vi "CSConnect.UpdateAllVoltages.vi"(0 "i ref in":refnum<vi>, 2 "In-channel number":i32, 3 "In-Voltage":dbl, 5 "error in (no error)":errorcluster) -> (14 "i ref out":refnum<vi>, 19 "error out":errorcluster)   [LabVIEW 2014, in "CSConnect.lvlib"]
doc: "Updates all voltages. This VI should be executed in ProcCases by the User. The idea is to only the \"Out\"-Voltages that need to be updated.\n\nLicense Agreement for this software:\n\nCopyright (C)\nGesellschaft für Schwerionenforschung, GSI\nPlanckstr. 1\n64291 Darmstadt\nGermany\n\nContact: D.Beck@gsi.de \n\nThis program is free software; you can redistribute it and/or modify it under the terms of the \nGNU General Public License as published by the Free Software Foundation; either version 2 of \nthe license, or (at your option) any later version.\n\nThis program is distributed in the hope that it will be useful, but WITHOUT ANY WARRANTY; \nwithout even the implied warranty of MERCHANTABILITY or FITNESS FOR A PARTICULAR PURPOSE. See the GNU General License for more details (http://www.gnu.org).\n\nGesellschaft für Schwerionenforschung, GSI\nPlanckstr. 1, 64291 Darmstadt, Germany\nFor all questions and ideas contact: M.Richter@gsi.de, H.Brand@gsi.de or D.Beck@gsi.de.\nLast update: 16-JUN-2004"
uses:
  CSConnect.lvlib
  CSCore/CSSystem/CoreLib/CoreLib.int 2 byte array.vi
  CSCore/CSSystem/CoreLib/CoreLib.double 2 byte array.vi
  CSCore/BaseProcess/BaseProcess.lvlib
  CSCore/CSSystem/CoreLib/CoreLib.lvlib
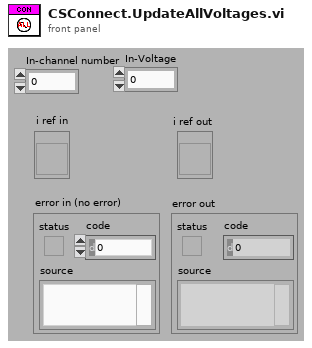
[diagram p1: front panel]
types:
  T1 = typedef "CSConnect.lvlib/CSConnect.i attribute.ctl" = cluster{"In-Array":cluster{"Alias":string, "Value":dbl, "neededOuts":bool[]}[], "Out-Array":cluster{"ObjectName":string, "VoltFunctionName":string, "OnOffFunctionName":string, "Channel":string, "Calculation-Formula":string}[], "OutChannelsID":i32, "InOutMatrixID":i32}
  T2 = cluster{"ObjectName":string, "VoltFunctionName":string, "OnOffFunctionName":string, "Channel":string, "Calculation-Formula":string}[]
  T3 = cluster{"Alias":string, "Value":dbl, "neededOuts":bool[]}[]
  T4 = cluster{"Alias":string, "Value":dbl, "neededOuts":bool[]}
  T5 = typedef "CoreDefs.rawDataType.ctl" = i8[]
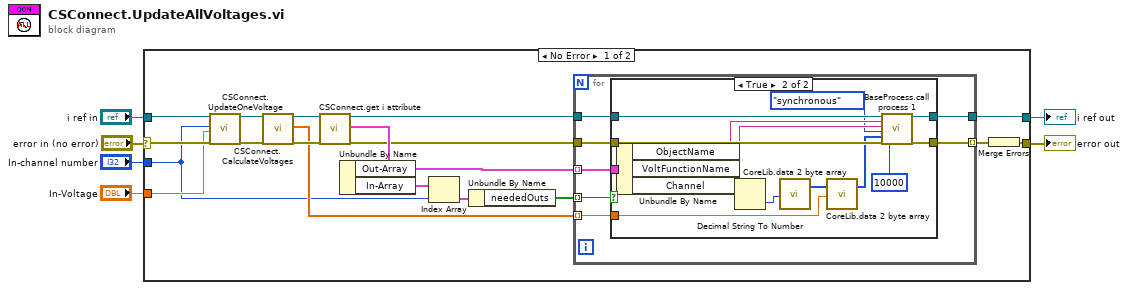
[diagram p0: block diagram]
diagram:
  n1 = case shown="No Error" "error in (no error)" {
    selector: "error in (no error)" -> [w24 w49]
    tunnel: [w12 w49] -> w6
    tunnel: [w13 w50] -> w4
    tunnel: "i ref in" -> [w25 w50]
    tunnel: "In-channel number" -> [w9 _]
    tunnel: "In-Voltage" -> [w23 _]
    frame No Error {
      n2 = call "CSConnect.UpdateOneVoltage.vi"("i ref in"=w25, "In-channel number"=w9, "In-Voltage"=w23, "error in (no error)"=w24) -> ("i ref out"=w22:refnum<vi>, "error out"=w21:errorcluster)  [unwired: 14 in]
      n3 = call "CSConnect.CalculateVoltages.vi"("i ref in"=w22, "error in (no error)"=w21) -> ("i ref out"=w19:refnum<vi>, "Array Out-Voltages"=w11:dbl[], "error out"=w20:errorcluster)  [unwired: 15 in]
      n4 = call "CSConnect.get i attribute.vi"("i ref in"=w19, "error in (no error)"=w20) -> ("i ref out"=w16:refnum<vi>, "i attribute"=w18:T1, "error out"=w15:errorcluster)  [unwired: 15 in]
      n5 = Unbundle By Name(w18) -> ("Out-Array"=w17:T2, "In-Array"=w10:T3)
      n6 = Index Array(array=w10, index=w9) -> (element=w8:T4)
      n7 = Unbundle By Name(w8) -> ("neededOuts"=w7:bool[])
      n8 = for {
        tunnel: w17 -> [w28] mode=indexing
        tunnel: w16 -> [w32]
        tunnel: w15 -> [w31]
        tunnel: [w30] -> w14 mode=indexing
        tunnel: [w29] -> w13
        tunnel: w11 -> [w27] mode=indexing
        tunnel: w7 -> [w26] mode=indexing
        n9 = case shown="True" w26 {
          tunnel: w32 -> [w34 w48]
          tunnel: w31 -> [w33 w47]
          tunnel: [w33 w46] -> w30
          tunnel: [w34 w45] -> w29
          tunnel: w28 -> [_ w43]
          tunnel: w27 -> [_ w39]
          frame False {
          }
          frame True {
            n10 = Unbundle By Name(w43) -> ("ObjectName"=w42:string, "VoltFunctionName"=w41:string, "Channel"=w36:string)
            n11 = Decimal String To Number(string=w36) -> (number=w35:i32)  [unwired: 2 in, 1 out]
            n12 = call-poly "CoreLib.data 2 byte array.vi"("i32"=w35) -> ("byteArray out"=w40:T5)  [unwired: 18 in]
            n13 = call-poly "CoreLib.data 2 byte array.vi"("byteArray"=w40, "f64"=w39) -> ("byteArray out"=w38:T5)  [unwired: 17 in]
            n14 = call "BaseProcess.call process 1.vi"("i ref in"=w48, "Object"=w42, "Selector"=w41, "CallType"=enum16{"simple", "synchronous", "asynchronous"}."synchronous", "Data"=w38, "error in (no error)"=w47, "timeout (ms)"=10000) -> ("i ref out"=w45:refnum<vi>, "error out"=w46:errorcluster)  [unwired: 10 in, 1 out]
          }
        }
      }
      n15 = Merge Errors(w14) -> (w12:errorcluster)
    }
    frame Error {
    }
  }
  "error out" <- w6
  "i ref out" <- w4
